vi "Chapter-One.vi"() -> ()   [LabVIEW 2023]
uses:
  MQTT-Server/MQTT-Server/MQTT-Server.lvclass
  MQTT-Client/MQTT-Client/MQTT-Client.lvclass
  <vilib>/ActorFramework/Message Enqueuer/Message Enqueuer.lvclass
  MQTT-Client/MQTT-Client/MQTT-Client.lvclass/MQTT-Client.ctl
  <vilib>/ActorFramework/Message Enqueuer/Message Enqueuer.lvclass/Message Enqueuer.ctl
  <vilib>/ActorFramework/Message Enqueuer/Enqueue.vi
  <vilib>/ActorFramework/Stop Msg/Stop Msg.lvclass
  <vilib>/ActorFramework/Message Priority Queue/Priority Enqueue.vi
  <vilib>/ActorFramework/Actor/Actor.lvclass
panel:
  in  "Client":i32 min=0 step=1
  in  "Server":bool
  in  "Stop":bool
  # "Client"
  # "Server"
  # "Demo"
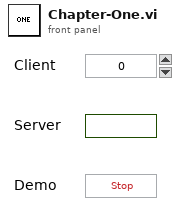
[diagram p1: front panel]
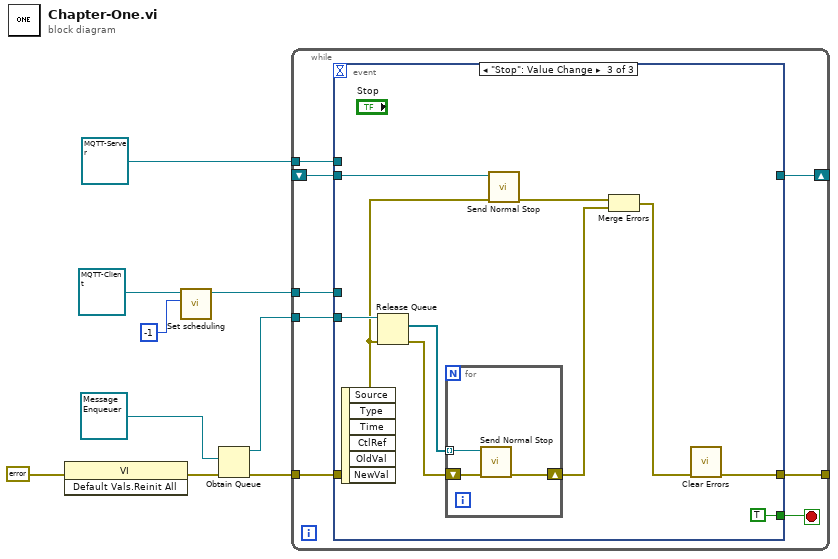
[diagram p0: block diagram]
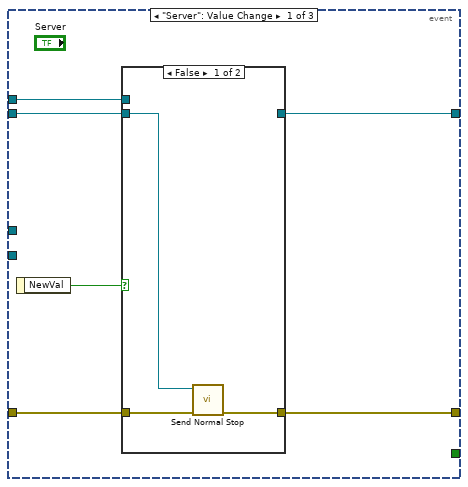
[diagram p2: hidden frame]
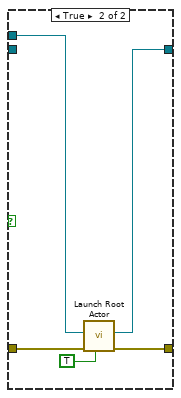
[diagram p3: hidden frame]
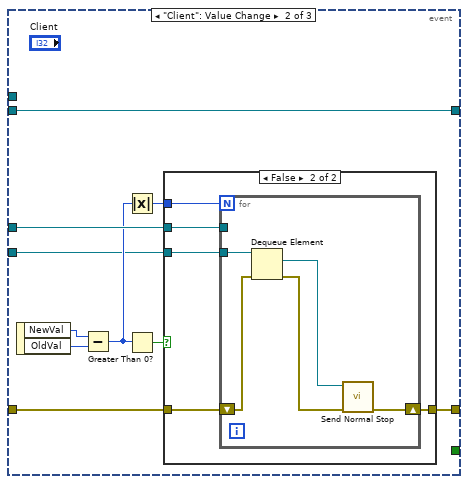
[diagram p4: hidden frame]
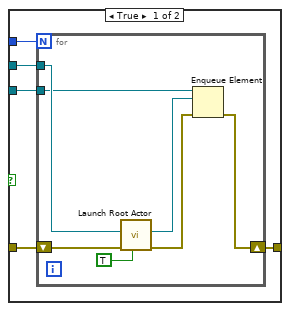
[diagram p5: hidden frame]
diagram:
  n1 = invoke class="VI" method="Default Vals.Reinit All"(error in=errorcluster {"status"=FALSE, "code"=0, "source"=""} ("error in (no error)")) -> (error out=w1:errorcluster)  [unwired: 2 in, 2 out]
  n2 = call "Set scheduling.vi"("scheduling"=-1, "MQTT-Client in"=refnum<class "MQTT-Client.lvclass"> refnum ("MQTT-Client.lvlib:MQTT-Client.lvclass")) -> ("MQTT-Client out"=w4:refnum<class "MQTT-Client.lvclass">)  [unwired: 8 in, 1 out]
  n3 = Obtain Queue(element data type=refnum<class "Message Enqueuer.lvclass"> refnum ("Actor's Enqueuer"), error in (no error)=w1) -> (queue out=w6:refnum<queue>, error out=w8:errorcluster)  [unwired: 3 in, 1 out]
  n4 = while {
    tunnel: refnum<class "MQTT-Server.lvclass"> refnum ("MQTT-Server.lvlib:MQTT-Server.lvclass") -> [w17]
    tunnel: w4 -> [w16]
    tunnel: w8 -> [w15]
    tunnel: [w14] -> _
    shift-right: [w13] -> _
    shift-left: _ -> [w12]
    tunnel: w6 -> [w11]
    stop <- w10 stop-if-true
    n5 = event shown="[2] \"Stop\": Value Change" {
      selector: _ -> [_ _ _]
      dyn-events: _ -> [_ _ _]
      timeout: _ -> [_ _ _]
      tunnel: w17 -> [w23 _ _]
      tunnel: w16 -> [_ w38 _]
      tunnel: w15 -> [w22 w37 w70]
      tunnel: [w21 w33 w65] -> w14
      tunnel: [w20 w41 _] -> w13
      tunnel: w12 -> [w19 w41 w69]
      tunnel: w11 -> [_ w34 w73]
      tunnel: [_ _ TRUE] -> w10
      event "Server": Value Change {
        n6 = event-data() -> ("NewVal"=w18:bool)  [unwired: 1 in]
        n7 = case shown="False" w18 {
          tunnel: w23 -> [_ w31]
          tunnel: w22 -> [w25 w30]
          tunnel: [w24 w28] -> w21
          tunnel: [_ w27] -> w20
          tunnel: w19 -> [w26 _]
          frame False {
            n8 = call <vilib>:"Send Normal Stop.vi"("error in (no error)"=w25, "Message Enqueuer"=w26) -> ("error out"=w24:errorcluster)  [unwired: 9 in]
          }
          frame True {
            n9 = call <vilib>:"Launch Root Actor.vi"("Open Actor Core front panel? (F)"=TRUE, "error in (no error)"=w30, "Actor"=w31) -> ("error out"=w28:errorcluster, "Actor's Enqueuer"=w27:refnum<class "Message Enqueuer.lvclass">)  [unwired: 7 in]
          }
        }
      }
      event "Client": Value Change {
        n10 = event-data() -> ("NewVal"=w40:i32, "OldVal"=w39:i32)  [unwired: 1 in]
        n11 = Subtract(x=w40, y=w39) -> (x-y=w36:i32)
        n12 = Absolute Value(x=w36) -> (abs(x)=w35:i32)
        n13 = Greater Than 0?(x=w36) -> (x > 0?=w32:bool)
        n14 = case shown="False" w32 {
          tunnel: w38 -> [w46 w58]
          tunnel: w37 -> [w45 w57]
          tunnel: w35 -> [w44 w56]
          tunnel: w34 -> [w43 w55]
          tunnel: [w42 w54] -> w33
          frame True {
            n15 = for {
              N: w44 -> [_]
              tunnel: w46 -> [w52]
              shift-right: [w47] -> w42
              shift-left: w45 -> [w53]
              tunnel: w43 -> [w50]
              n16 = call <vilib>:"Launch Root Actor.vi"("Open Actor Core front panel? (F)"=TRUE, "error in (no error)"=w53, "Actor"=w52) -> ("error out"=w49:errorcluster, "Actor's Enqueuer"=w48:refnum<class "Message Enqueuer.lvclass">)  [unwired: 7 in]
              n17 = Enqueue Element(queue=w50, element=w48, error in (no error)=w49) -> (error out=w47:errorcluster)  [unwired: 1 in, 2 out]
            }
          }
          frame False {
            n18 = for {
              N: w56 -> [_]
              tunnel: w58 -> [_]
              shift-right: [w59] -> w54
              shift-left: w57 -> [w62]
              tunnel: w55 -> [w63]
              n19 = Dequeue Element(queue=w63, error in (no error)=w62) -> (element=w61:refnum<class "Message Enqueuer.lvclass">, error out=w60:errorcluster)  [unwired: 1 in, 2 out]
              n20 = call <vilib>:"Send Normal Stop.vi"("error in (no error)"=w60, "Message Enqueuer"=w61) -> ("error out"=w59:errorcluster)  [unwired: 9 in]
            }
          }
        }
      }
      event "Stop": Value Change {
        n21 = event-data() -> ()  [unwired: 1 in, 6 out]
        n22 = Release Queue(queue=w73, error in (no error)=w70) -> (remaining elements=w71:refnum<class "Message Enqueuer.lvclass">[], error out=w72:errorcluster)  [unwired: 1 in, 1 out]
        n23 = for {
          tunnel: w71 -> [w75] mode=indexing
          shift-right: [w74] -> w68
          shift-left: w72 -> [w76]
          n24 = call <vilib>:"Send Normal Stop.vi"("error in (no error)"=w76, "Message Enqueuer"=w75) -> ("error out"=w74:errorcluster)  [unwired: 9 in]
        }
        n25 = call <vilib>:"Send Normal Stop.vi"("error in (no error)"=w70, "Message Enqueuer"=w69) -> ("error out"=w67:errorcluster)  [unwired: 9 in]
        n26 = Merge Errors(w67, w68) -> (w66:errorcluster)
        n27 = call <vilib>:"Clear Errors.vi"("error in (no error)"=w66) -> ("error out"=w65:errorcluster)  [unwired: 5 in, 1 out]
      }
    }
  }
